vi "Config Measure Preset Normal.vi"(0 "VISA resource name":refnum<visa-resource-name>, 5 "Preset Pattern (0: Clear)":u16(ring) items=["Clear", "Normal", "Integrate"], 11 "error in (no error)":errorcluster) -> (4 "VISA resource name out":refnum<visa-resource-name>, 15 "error out":errorcluster)   [LabVIEW 2016, in "Yokogawa WT200 Series.lvlib"]
doc: "This VI sends the Normal Preset Measurement Configuration command to the WT200 Series."
uses:
  Yokogawa WT200 Series.lvlib
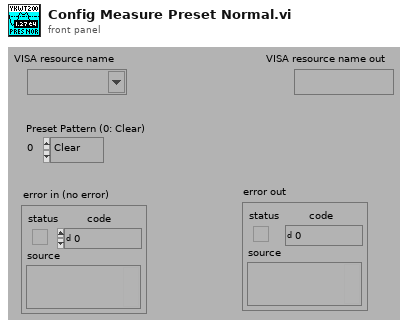
[diagram p1: front panel]
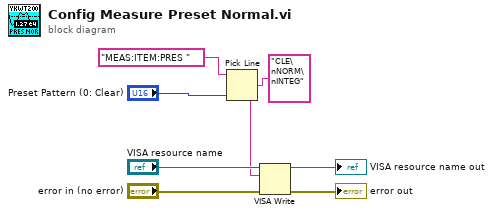
[diagram p0: block diagram]
diagram:
  n1 = Pick Line(string ("")="MEAS:ITEM:PRES ", multi-line string="CLE\nNORM\nINTEG", line index="Preset Pattern (0: Clear)") -> (output string=w1:string)
  n2 = VISA Write(VISA resource name="VISA resource name", write buffer=w1, error in (no error)="error in (no error)") -> (VISA resource name out=→"VISA resource name out":refnum<visa-resource-name>, error out=→"error out":errorcluster)  [unwired: 1 out]
